vi "Is Over-Range Core.vi"(8 "error in (no error)":errorcluster, 10 "measurement value":dbl format="%^.2e", 11 "IVI_DMM_Delayed in":refnum<class "IVI_DMM_Delayed.lvclass">) -> (0 "error out":errorcluster, 2 "is over-range":bool, 3 "IVI_DMM_Delayed out":refnum<class "IVI_DMM_Delayed.lvclass">)   [LabVIEW 2015, in "IVI_DMM.lvlib" / "IVI_DMM_Delayed.lvclass"]
doc: "This VI takes a measurement value that you obtain from either the Read or Fetch VIs and determines if the value is a valid measurement value or a value indicating that an over-range condition occurred. \n\nNotes:\n\n(1) If an over-range condition occurs, the measurement value contains an IEEE defined NaN (Not a Number) value indicating that an over-range condition occurred.\n\n(2) This VI does not check the instrument status."
uses:
  IVI_DMM_Delayed.lvclass
  IVI_DMM_Delayed.lvclass/IVI_DMM_Delayed.ctl
  IVI_DMM/IVI_DMM.lvclass
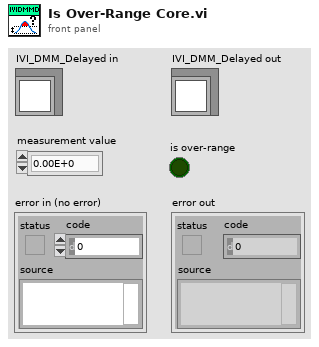
[diagram p1: front panel]
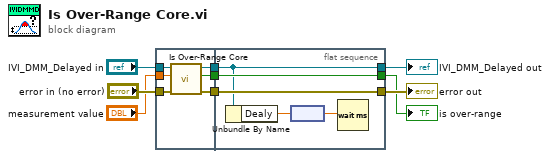
[diagram p0: block diagram]
diagram:
  n1 = flat-sequence {
    tunnel: "error in (no error)" -> [w12]
    tunnel: "measurement value" -> [w11]
    tunnel: "IVI_DMM_Delayed in" -> [w10]
    tunnel: [w15] -> w3
    tunnel: [w14] -> w2
    tunnel: [w13] -> w1
    tunnel: [w16] -> w7
    tunnel: [w20] -> w8
    tunnel: [w17] -> w9
    tunnel: w3 -> [w17]
    tunnel: w2 -> [w20]
    tunnel: w1 -> [w16]
    frame #0 {
      n2 = call-parent "Is Over-Range Core.vi"("error in (no error)"=w12, "measurement value"=w11, "IVI_DMM in"=w10) -> ("error out"=w15:errorcluster, "is over-range"=w14:bool, "IVI_DMM out"=w13:refnum<class "IVI_DMM_Delayed.lvclass">)  [unwired: 6 in]
    }
    frame #1 {
      n3 = Unbundle By Name(w16) -> ("Dealy"=w18:dbl[unit])
      n4 = node(w18) -> (w19:dbl)
      n5 = Wait (ms)(milliseconds to wait=w19) -> ()  [unwired: 1 out]
    }
  }
  "error out" <- w9
  "IVI_DMM_Delayed out" <- w7
  "is over-range" <- w8
